vi "TEMPLATE_Regular_Return.vi"(8 "Error In":errorcluster, 11 "QObject In":refnum<class "QObject.lvclass">) -> (0 "Error Out":errorcluster, 2 "Value":string, 3 "QObject Out":refnum<class "QObject.lvclass">)   [LabVIEW 2013, in "Template.lvlib" / "QObject.lvclass"]
uses:
  QObject.lvclass
  QObject.lvclass/QObject.ctl
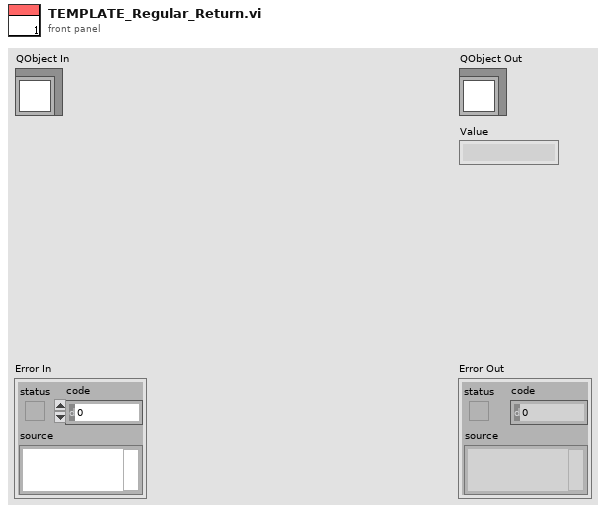
[diagram p1: front panel]
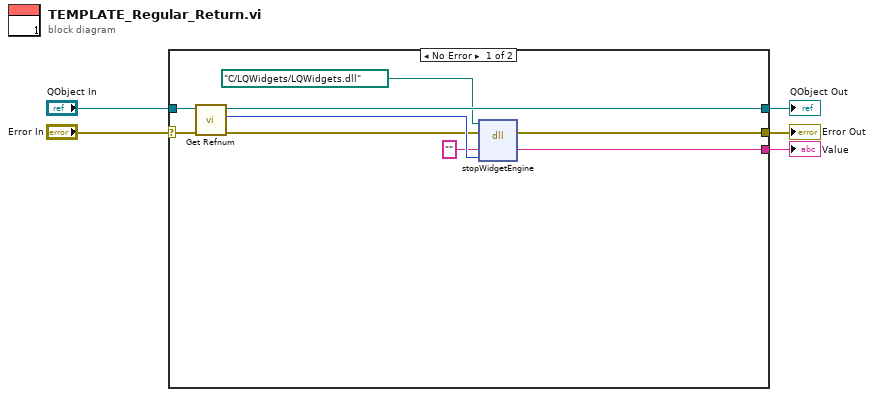
[diagram p0: block diagram]
diagram:
  n1 = case shown="No Error" "Error In" {
    selector: "Error In" -> [w10 w16]
    tunnel: [w14 w16] -> w4
    tunnel: [w12 w15] -> w2
    tunnel: "QObject In" -> [w13 w15]
    tunnel: [w7 _] -> w1
    frame No Error {
      n2 = call "Get Refnum.vi"("error in (no error)"=w10, "QObject in"=w13) -> ("error out"=w9:errorcluster, "Refnum"=w11:u32, "QObject out"=w12:refnum<class "QObject.lvclass">)  [unwired: 7 in]
      n3 = dll-call lib="?" fn="stopWidgetEngine"(path in=path "C:/LQWidgets/LQWidgets.dll", error in=w9, "retVal"="", "obj"=w11) -> (error out=w14:errorcluster, "retVal"=w7:string)  [unwired: 3 in, 1 out]
    }
    frame Error {
    }
  }
  "Error Out" <- w4
  "QObject Out" <- w2
  "Value" <- w1
